vi "CoordToAxesXY.vi"(8 "error in (no error)":errorcluster, 10 "Coords":T1, 11 "IntensityGraph in":refnum<vi>) -> (0 "error out":errorcluster, 2 "XY":cluster{"X":dbl, "Y":dbl}, 3 "IntensityGraph out":refnum<vi>)   [LabVIEW 2023]
doc: "Translate screen coordinates to graph XY axes values coordinates"
uses:
  <vilib>/Utility/miscctls.llb/LVPoint32TypeDef.ctl
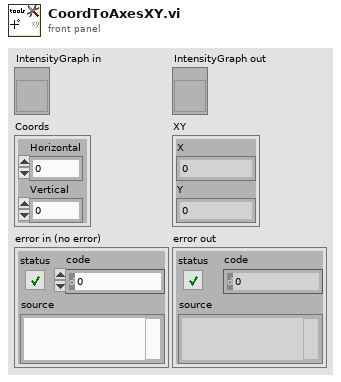
[diagram p1: front panel]
types:
  T1 = typedef "LVPoint32TypeDef.ctl" = cluster{"Horizontal":i32, "Vertical":i32}
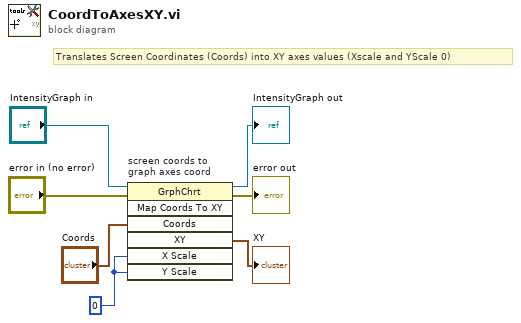
[diagram p0: block diagram]
diagram:
  w4 = 0 ("X Scale")
  # "Translates Screen Coordinates (Coords) into XY axes values (Xscale and YScale 0)"
  n1 = invoke on="screen coords to \ngraph axes coord" class="GrphChrt" method="Map Coords To XY"(reference="IntensityGraph in", error in="error in (no error)", "Coords"="Coords", "X Scale"=w4, "Y Scale"=w4) -> (reference out=→"IntensityGraph out":refnum<vi>, error out=→"error out":errorcluster, "XY"=→"XY":cluster{"X":dbl, "Y":dbl})  [unwired: 2 in, 4 out]
